vi "BRig_Host_v0,51.vi"() -> ()   [LabVIEW 2014]
uses:
  BRig_Host__global__stopHost.vi
  <vilib>/WebDAVClient/NI_WebDAV.lvlib
  <vilib>/WebDAVClient/Advanced/SessionHandle.ctl
  <vilib>/Utility/file.llb/Write To Spreadsheet File (DBL).vi
panel:
  out "writeError":bool
  out "error IO":errorcluster
  out "error_loopP_loadSettings":errorcluster caption="error out"
  out "testCmdList":u16[][](array[numeric])
  in  "ClosedLoop":bool
  in  "module":string=" module1 "
  in  "input_updateTrial_subsequent":u16
  in  "input_updateTrial_first":u16
  in  "input_forceUpdate":bool
  in  "ClosedLoop":u16[](array[numeric])
  in  "testNewLaserSettings":bool
  in  "LoadSettings":bool
  in  "DisplayNumber":u16
  out "XY Graph":cluster{u16[], u16[]}[](graph)
  in  "threshold_2":u16=600
  in  "threshold_1":u16=300
  in  "Port (F=A/B, T=C)":bool
  out "I_ExpRun":bool
  out "TCP_connection":bool
  in  "stopHost":bool
  # "Port Switch\nToggle TRUE if debugging"
  # "# Trials Displayed\n( 0 = all )"
  # "Selection\nTime Thresholds"
  # "Exp Run\nIn Progress"
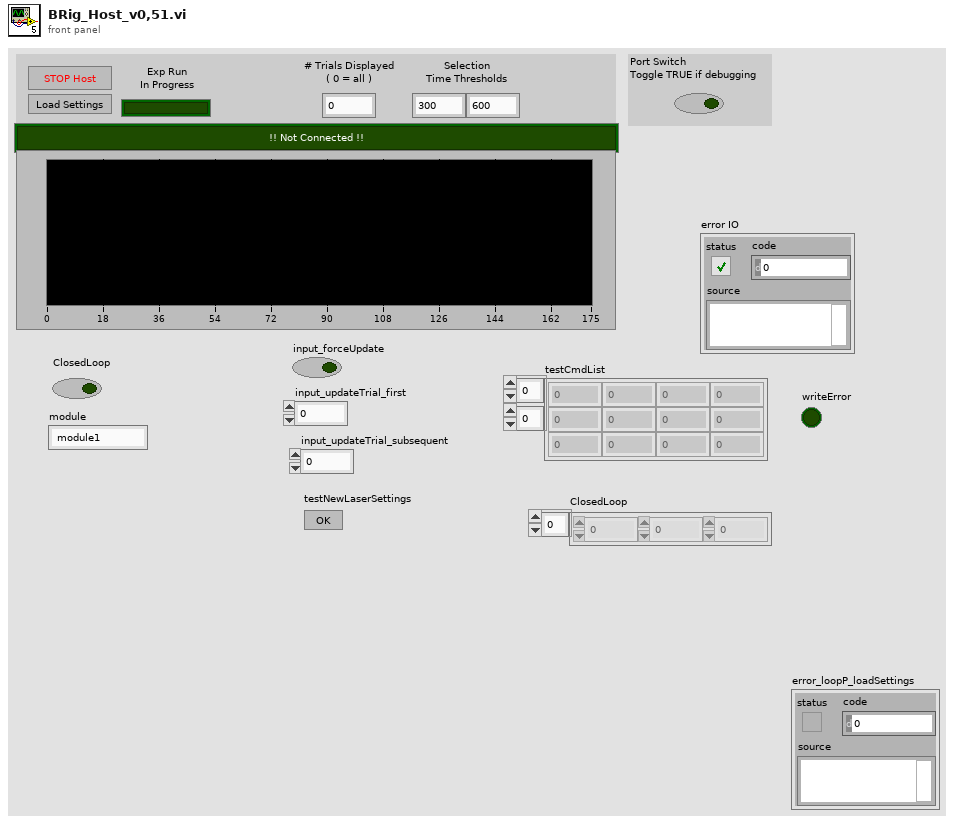
[diagram p1: front panel]
types:
  T1 = typedef "NI_WebDAV.lvlib/SessionHandle.ctl" = refnum<k1>
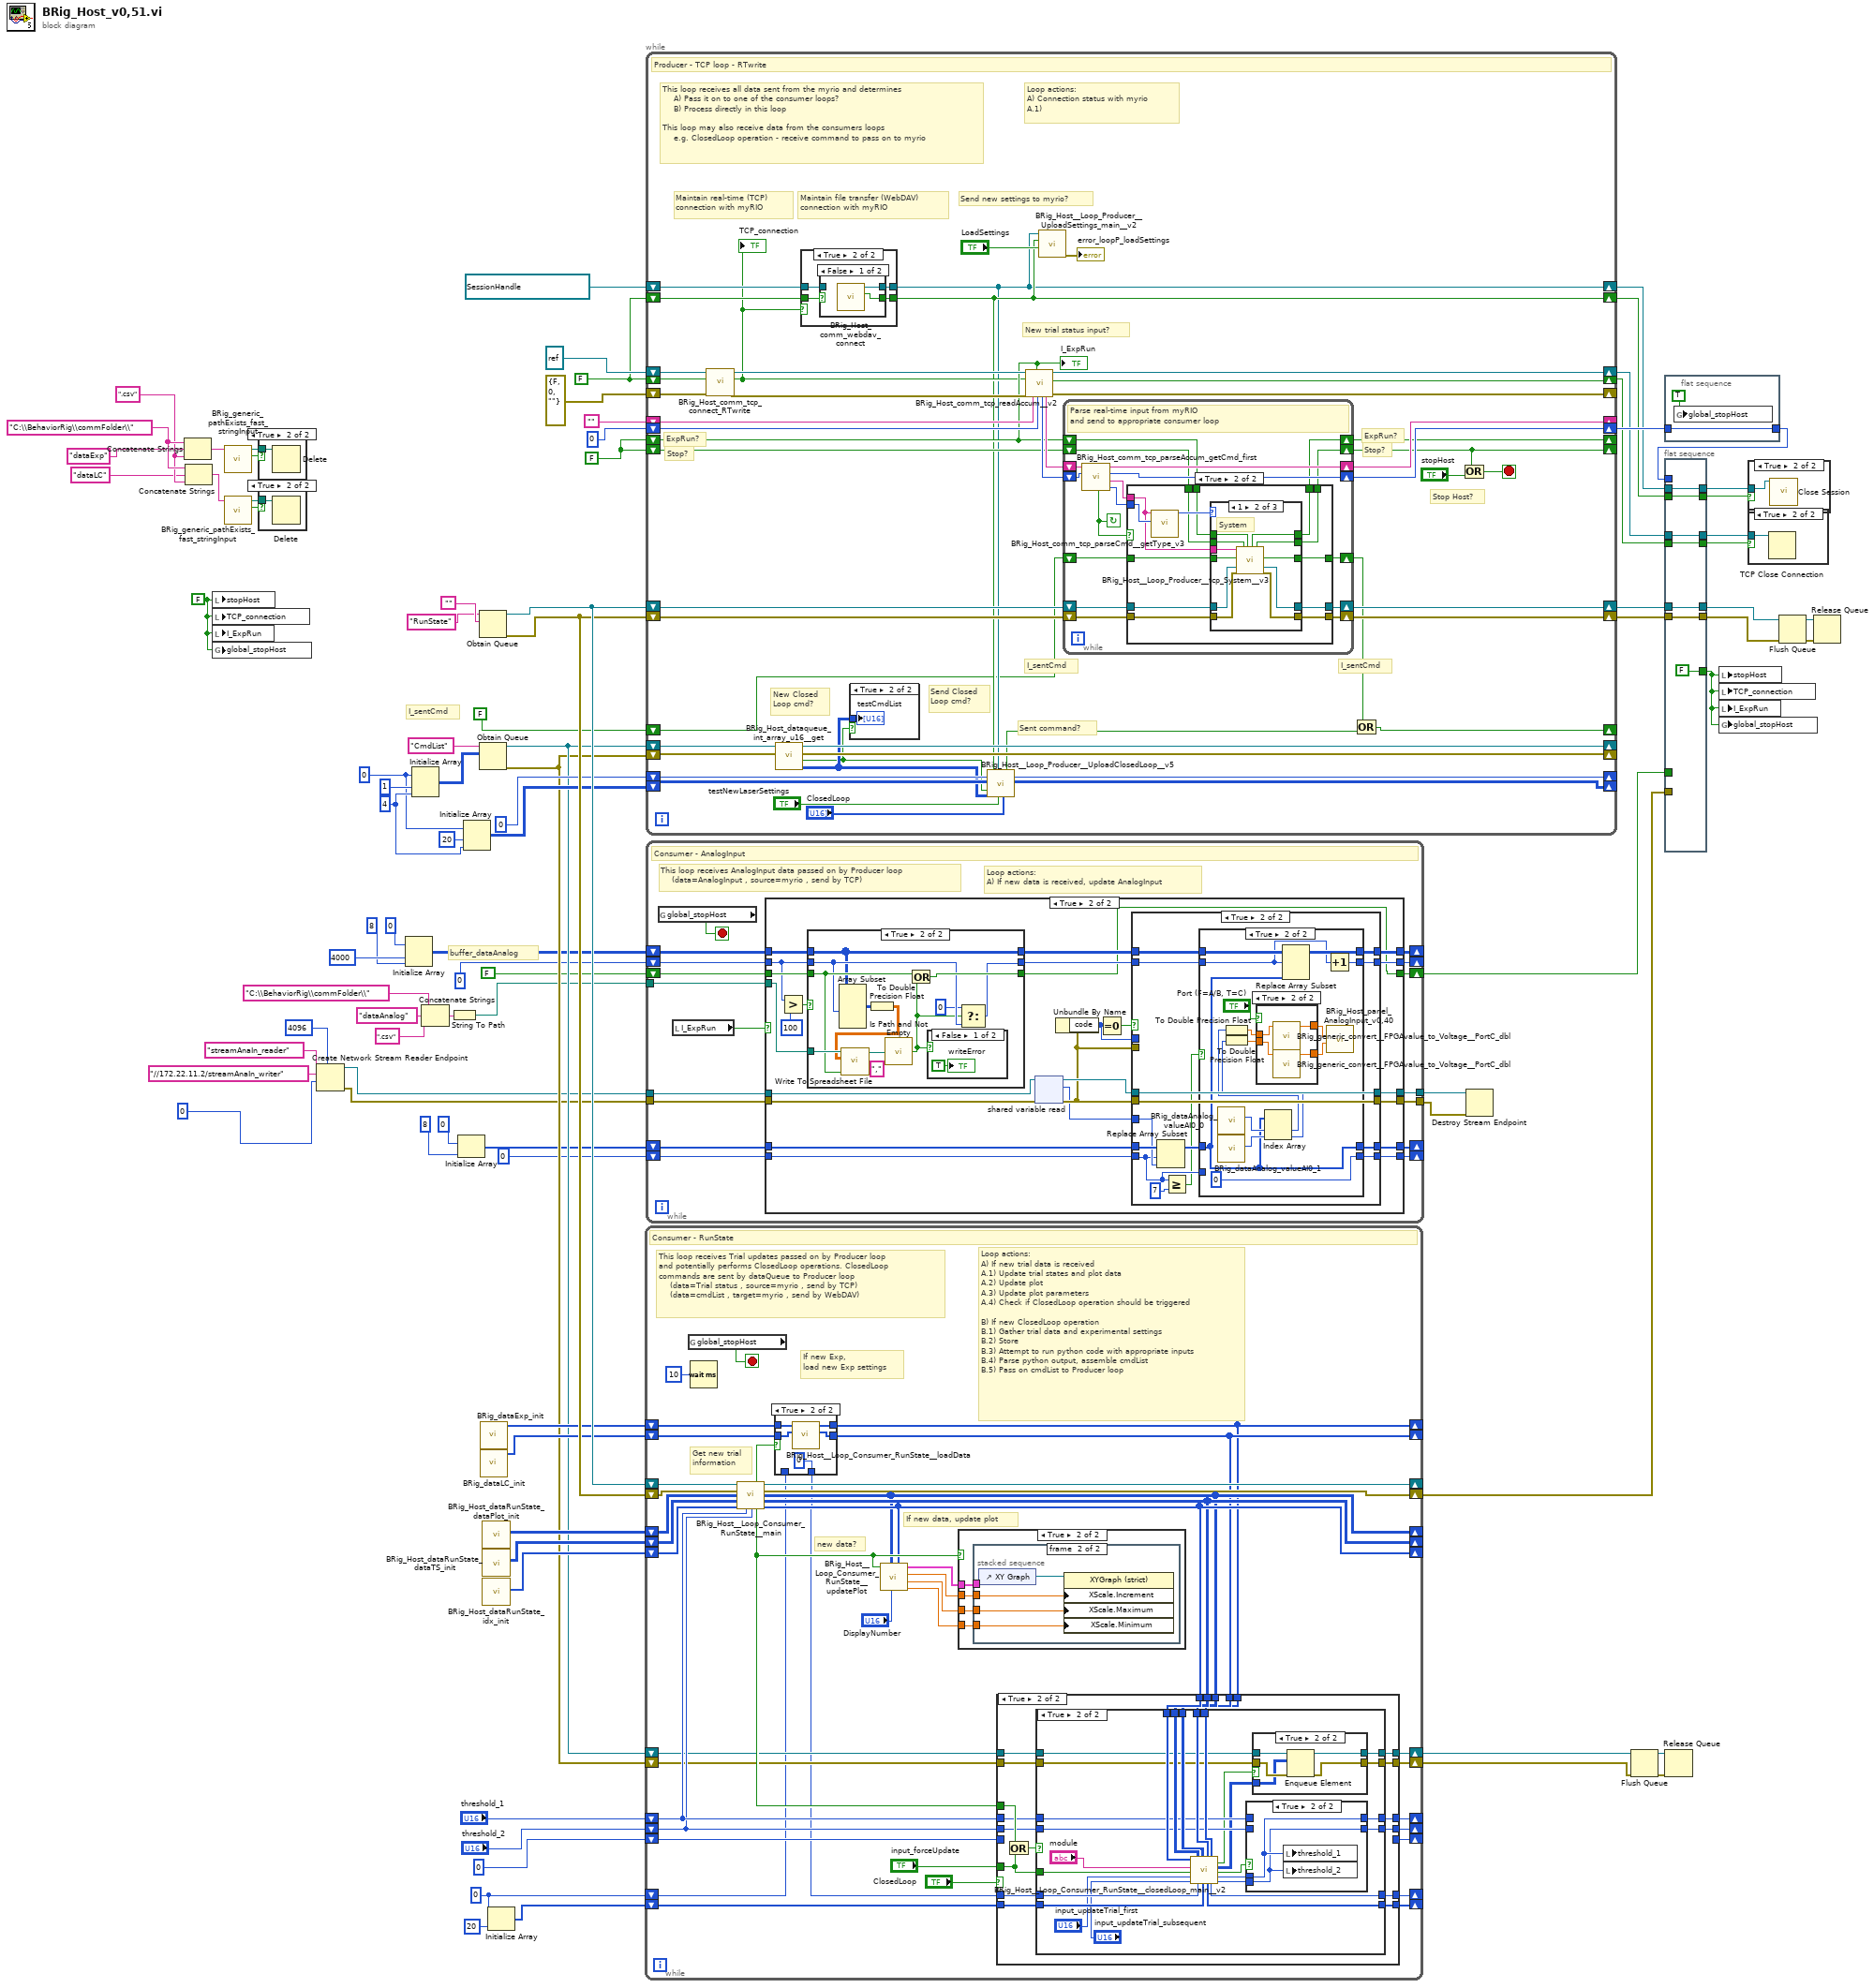
[diagram p0: block diagram]
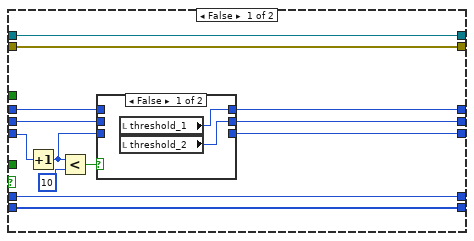
[diagram p6: hidden frame]
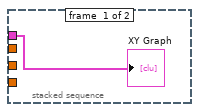
[diagram p13: hidden frame]
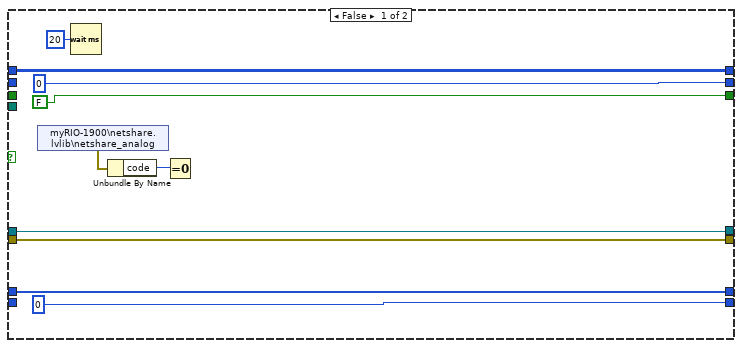
[diagram p14: hidden frame]
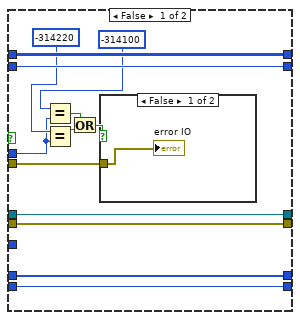
[diagram p15: hidden frame]
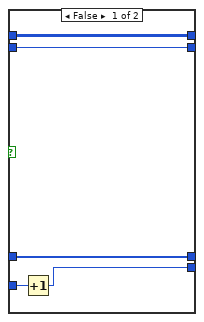
[diagram p17: hidden frame]
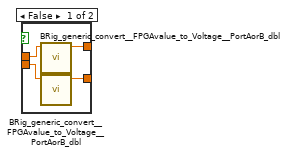
[diagram p18: hidden frame]
diagram:
  w25 = u16 0 ("element")
  w26 = 4 ("dimension size")
  w42 = u16 0
  w54 = ".csv" ("string")
  w55 = "C:\\BehaviorRig\\commFolder\\"
  w67 = T1 refnum items=["Session NI_WebDAV"] ("session handle")
  w85 = FALSE ("stopHost")
  w86 = FALSE
  w68 = FALSE
  # "buffer_dataAnalog"
  # "I_sentCmd"
  n1 = Concatenate Strings(w55, "dataExp" ("string"), w54) -> (w49:string)
  n2 = Concatenate Strings(w55, "dataLC" ("string"), w54) -> (w46:string)
  n3 = local write "stopHost"(w85) -> ()
  n4 = local write "TCP_connection"(w85) -> ()
  n5 = local write "I_ExpRun"(w85) -> ()
  n6 = global write "BRig_Host__global__stopHost.vi" "global_stopHost"(w85) -> ()
  n7 = call "BRig_generic_pathExists_fast_stringInput.vi"("input_filePath"=w49) -> ("output_Iexist"=w51:bool, "output_filePath"=w50:path)  [unwired: 8 in, 1 out]
  n8 = call "BRig_generic_pathExists_fast_stringInput.vi"("input_filePath"=w46) -> ("output_Iexist"=w47:bool, "output_filePath"=w48:path)  [unwired: 8 in, 1 out]
  n9 = case shown="True" w51 {
    tunnel: w50 -> [_ w91]
    frame False {
    }
    frame True {
      n10 = Delete(path (use dialog)=w91) -> ()  [unwired: 4 in, 3 out]
    }
  }
  n11 = case shown="True" w47 {
    tunnel: w48 -> [_ w92]
    frame False {
    }
    frame True {
      n12 = Delete(path (use dialog)=w92) -> ()  [unwired: 4 in, 3 out]
    }
  }
  n13 = Create Network Stream Reader Endpoint(7:4096 ("reader buffer size"), 9:u16 0 ("element"), 10:"//172.22.11.2/streamAnaIn_writer" ("writer url"), 11:"streamAnaIn_reader" ("reader name")) -> (0:w9:errorcluster, 3:w10:refnum<k21>)  [unwired: 3 in]
  n14 = Initialize Array(u16 0 ("element"), 4000 ("dimension size"), 8 ("dimension size")) -> (w21:u16[][])
  n15 = Initialize Array(w25, 1 ("dimension size"), w26) -> (w37:u16[][])
  n16 = Concatenate Strings("C:\\BehaviorRig\\commFolder\\" ("string"), "dataAnalog" ("input_filename"), ".csv" ("string")) -> (w18:string)
  n17 = String To Path(string=w18) -> (path=w15:path)
  n18 = Initialize Array(u16 0 ("element"), 8 ("dimension size")) -> (w2:u16[])
  n19 = Initialize Array(w25, 20 ("dimension size"), w26) -> (w56:u16[][])
  n20 = Obtain Queue(name (unnamed)="RunState", element data type="") -> (queue out=w77:refnum<queue>, error out=w76:errorcluster)  [unwired: 3 in, 1 out]
  n21 = Obtain Queue(name (unnamed)="CmdList", element data type=w37) -> (queue out=w36:refnum<queue>, error out=w35:errorcluster)  [unwired: 3 in, 1 out]
  n22 = call "BRig_dataExp_init.vi"() -> ("output_dataExp"=w45:u16[])  [unwired: 11 in]
  n23 = call "BRig_dataLC_init.vi"() -> ("output_dataLC"=w44:u16[])  [unwired: 11 in]
  n24 = call "BRig_Host_dataRunState_dataPlot_init.vi"() -> ("output_dataPlot"=w73:u16[][])  [unwired: 11 in]
  n25 = call "BRig_Host_dataRunState_dataTS_init.vi"() -> ("output_dataTS"=w72:u16[][])  [unwired: 11 in]
  n26 = call "BRig_Host_dataRunState_idx_init.vi"() -> ("output_idx"=w71:i32[])  [unwired: 11 in]
  n27 = Initialize Array(w42, 20 ("dimension size")) -> (w40:u16[])
  n28 = while {
    shift-right: [w124] -> _
    shift-left: w77 -> [w125]
    shift-right: [w122] -> w30
    shift-left: w76 -> [w123]
    shift-right: [w105] -> _
    shift-left: w73 -> [w121]
    shift-right: [w106] -> _
    shift-left: w72 -> [w120]
    shift-right: [w107] -> _
    shift-left: w71 -> [w119]
    shift-right: [w115] -> _
    shift-left: "threshold_1" -> [w114]
    shift-right: [w113] -> _
    shift-left: "threshold_2" -> [w112]
    shift-right: [w103] -> _
    shift-left: w45 -> [w117]
    shift-right: [w104] -> _
    shift-left: w44 -> [w116]
    shift-right: [w97] -> _
    shift-left: w42 -> [w95]
    shift-right: [w109] -> _
    shift-left: u8 0 -> [w110]
    shift-right: [w96] -> _
    shift-left: w40 -> [w93]
    shift-right: [w100] -> w32
    shift-left: w36 -> [w102]
    shift-right: [w99] -> w31
    shift-left: w35 -> [w101]
    stop <- w132 stop-if-true
    # "Loop actions:\nA) If new trial data is received\nA.1) Update trial states and plot data\nA.2) Update plot\nA.3) Update plot parameters\nA.4) Check if ClosedLoop operation should be triggered\n\nB) If new ClosedLoop operation\nB.1) Gather trial data and experimental settings\nB.2) Store\nB.3) Attempt to run python code with appropriate inputs\nB.4) Parse python output, assemble cmdList\nB.5) Pass on cmdList to Producer loop"
    # "This loop receives Trial updates passed on by Producer loop\nand potentially performs ClosedLoop operations. ClosedLoop\ncommands are sent by dataQueue to Producer loop\n    (data=Trial status , source=myrio , send by TCP)\n    (data=cmdList , target=myrio , send by WebDAV)"
    # "If new data, update plot"
    # "If new Exp,\nload new Exp settings"
    # "new data?"
    # "Get new trial\ninformation"
    # "Consumer - RunState"
    n29 = global read "BRig_Host__global__stopHost.vi" "global_stopHost"() -> (w132:bool)
    n30 = Wait (ms)(milliseconds to wait=u32 10) -> ()  [unwired: 1 out]
    n31 = call "BRig_Host__Loop_Consumer_RunState__main.vi"("input_hDataQueue"=w125, "input_errorDataQueue"=w123, "input_dataPlot"=w121, "input_dataTS"=w120, "input_idx"=w119, "threshold_1"=w114, "threshold_2"=w112) -> ("output_ExpStart"=w118:bool, "output_hDataQueue"=w124:refnum<queue>, "output_errorDataQueue"=w122:errorcluster, "output_dataPlot"=w105:u16[][], "output_dataTS"=w106:u16[][], "output_updatePlot"=w108:bool, "output_idx"=w107:i32[])  [unwired: 2 in]
    n32 = case shown="True" w118 {
      tunnel: w117 -> [w216 w218]
      tunnel: [w216 w221] -> w103
      tunnel: w116 -> [w215 w219]
      tunnel: [w215 w220] -> w104
      tunnel: w95 -> [w214 _]
      tunnel: [w214 u16 0] -> w94
      frame False {
      }
      frame True {
        n33 = call "BRig_Host__Loop_Consumer_RunState__loadData.vi"("input_dataLC"=w219, "input_dataExp"=w218) -> ("output_dataLC"=w220:u16[], "output_dataExp"=w221:u16[])  [unwired: 8 in]
      }
    }
    n34 = call "BRig_Host__Loop_Consumer_RunState__updatePlot.vi"("input_idx"=w107, "input_DisplayNumber"="DisplayNumber", "input_dataPlot"=w105, "input_updatePlot"=w108) -> ("output_X_min"=w128:dbl, "output_X_max"=w127:dbl, "output_X_inc"=w126:dbl, "XY Graph"=w129:cluster{u16[], u16[]}[])  [unwired: 4 in]
    n35 = case shown="True" w108 {
      tunnel: w129 -> [_ w225]
      tunnel: w128 -> [_ w224]
      tunnel: w127 -> [_ w223]
      tunnel: w126 -> [_ w222]
      frame False {
      }
      frame True {
        n36 = stacked-sequence {
          tunnel: w225 -> [w226 _]
          tunnel: w224 -> [_ w229]
          tunnel: w223 -> [_ w228]
          tunnel: w222 -> [_ w227]
          frame #0 {
            "XY Graph" <- w226
          }
          frame #1 {
            n37 = control-ref of="XY Graph"() -> (w230:refnum<vi>)
            n38 = property class="XYGraph (strict)"(reference=w230, "XScale.Increment"=w227, "XScale.Maximum"=w228, "XScale.Minimum"=w229) -> ()  [unwired: 1 in, 2 out]
          }
        }
      }
    }
    n39 = case shown="True" "ClosedLoop" {
      tunnel: [w140 w163] -> w115
      tunnel: w114 -> [w141 w164]
      tunnel: [w139 w161] -> w113
      tunnel: w112 -> [w142 w162]
      tunnel: w110 -> [w145 _]
      tunnel: [w138 _] -> w109
      tunnel: w94 -> [w136 w168]
      tunnel: [w136 w166] -> w97
      tunnel: w93 -> [w135 w167]
      tunnel: [w135 w165] -> w96
      tunnel: w108 -> [_ w170]
      tunnel: w107 -> [_ w160]
      tunnel: w106 -> [_ w159]
      tunnel: w105 -> [_ w158]
      tunnel: w104 -> [_ w157]
      tunnel: w103 -> [_ w156]
      tunnel: w102 -> [w134 w155]
      tunnel: w101 -> [w133 w154]
      tunnel: [w134 w153] -> w100
      tunnel: [w133 w152] -> w99
      tunnel: "input_forceUpdate" -> [_ w151]
      frame False {
        n40 = Increment(x=w145) -> (x+1=w137:u8)
        n41 = Less?(x=w137, y=u8 10) -> (x < y?=w143:bool)
        n42 = case shown="False" w143 {
          tunnel: w142 -> [_ w149]
          tunnel: w141 -> [_ w150]
          tunnel: [w147 w150] -> w140
          tunnel: [w146 w149] -> w139
          tunnel: [_ w148] -> w138
          tunnel: w137 -> [_ w148]
          frame False {
            n43 = local read "threshold_1"() -> (w147:u16)
            n44 = local read "threshold_2"() -> (w146:u16)
          }
          frame True {
          }
        }
      }
      frame True {
        n45 = Or(x=w170, y=w151) -> (x .or. y?=w169:bool)
        n46 = case shown="True" w169 {
          tunnel: w151 -> [_ w199]
          tunnel: w168 -> [w176 w202]
          tunnel: w167 -> [w175 w201]
          tunnel: [w176 w195] -> w166
          tunnel: [w175 w196] -> w165
          tunnel: w164 -> [w174 w189]
          tunnel: [w174 w185] -> w163
          tunnel: w162 -> [w173 w188]
          tunnel: [w173 w184] -> w161
          tunnel: w160 -> [_ w194]
          tunnel: w159 -> [_ w193]
          tunnel: w158 -> [_ w192]
          tunnel: w157 -> [_ w191]
          tunnel: w156 -> [_ w190]
          tunnel: w155 -> [w172 w182]
          tunnel: w154 -> [w171 w180]
          tunnel: [w172 w181] -> w153
          tunnel: [w171 w179] -> w152
          frame False {
          }
          frame True {
            n47 = call "BRig_Host__Loop_Consumer_RunState__closedLoop_main__v2.vi"("input_idx"=w194, "input_module"="module", "input_forceUpdate"=w199, "input_updateTrial_first"="input_updateTrial_first", "input_updateTrial_subsequent"="input_updateTrial_subsequent", "input_dataTS"=w193, "input_updateID"=w202, "input_dataPlot"=w192, "input_trialList"=w201, "input_dataLC"=w191, "input_dataExp"=w190) -> ("output_trialList"=w196:u16[], "output_updateID"=w195:u16, 15:"output_cmdList"=w177:bool, 16:"output_cmdList"=w178:u16[][], "output_thres"=w183:bool, "output_thres1"=w187:u16, "output_thres2"=w186:u16)  [unwired: 2 in]
            n48 = case shown="True" w183 {
              tunnel: w189 -> [w211 _]
              tunnel: w188 -> [w210 _]
              tunnel: w187 -> [_ w213]
              tunnel: w186 -> [_ w212]
              tunnel: [w211 w213] -> w185
              tunnel: [w210 w212] -> w184
              frame False {
              }
              frame True {
                n49 = local write "threshold_1"(w213) -> ()
                n50 = local write "threshold_2"(w212) -> ()
              }
            }
            n51 = case shown="True" w177 {
              tunnel: w182 -> [w204 w209]
              tunnel: [w204 w206] -> w181
              tunnel: w180 -> [w203 w208]
              tunnel: [w203 w205] -> w179
              tunnel: w178 -> [_ w207]
              frame False {
              }
              frame True {
                n52 = Enqueue Element(queue=w209, element=w207, error in (no error)=w208) -> (queue out=w206:refnum<queue>, error out=w205:errorcluster)  [unwired: 1 in, 1 out]
              }
            }
          }
        }
      }
    }
  }
  n53 = while {
    shift-right: [w257] -> w61
    shift-left: w68 -> [w277]
    shift-right: [w272] -> w62
    shift-left: refnum<k5> refnum ("output_hTCP") -> [w276]
    shift-right: [w271] -> _
    shift-left: errorcluster {"status"=FALSE, "code"=0, "source"=""} ("output_error") -> [w275]
    shift-right: [w266] -> _
    shift-left: "" ("input_strAccum") -> [w270]
    shift-right: [w265] -> w75
    shift-left: 0 ("input_count") -> [w269]
    shift-right: [w264] -> _
    shift-left: w86 -> [w242]
    shift-right: [w240] -> _
    shift-left: w86 -> [w262]
    shift-right: [w259] -> w81
    shift-left: w77 -> [w261]
    shift-right: [w258] -> w80
    shift-left: w76 -> [w260]
    shift-right: [w237] -> w66
    shift-left: w68 -> [w256]
    shift-right: [w236] -> w65
    shift-left: w67 -> [w255]
    shift-right: [w247] -> _
    shift-left: w56 -> [w248]
    shift-right: [w231] -> _
    shift-left: 0 -> [w249]
    shift-right: [w251] -> _
    shift-left: w36 -> [w253]
    shift-right: [w250] -> _
    shift-left: w35 -> [w252]
    shift-right: [w232] -> _
    shift-left: FALSE -> [w235]
    stop <- w239 stop-if-true
    # "Sent command?"
    # "I_sentCmd"
    # "I_sentCmd"
    # "Stop Host?"
    # "Send Closed\nLoop cmd?"
    # "New Closed\nLoop cmd?"
    # "New trial status input?"
    # "ExpRun?"
    # "Stop?"
    # "Loop actions:\nA) Connection status with myrio\nA.1)"
    # "This loop receives all data sent from the myrio and determines\n    A) Pass it on to one of the consumer loops?\n    B) Process directly in this loop\n\nThis loop may also receive data from the consumers loops\n    e.g. ClosedLoop operation - receive command to pass on to myrio"
    # "Send new settings to myrio?"
    # "ExpRun?"
    # "Stop?"
    # "Maintain real-time (TCP)\nconnection with myRIO"
    # "Maintain file transfer (WebDAV)\nconnection with myRIO"
    # "Producer - TCP loop - RTwrite"
    n54 = call "BRig_Host_comm_tcp_connect_RTwrite.vi"("input_error"=w275, "input_connected"=w277, "input_hTCP"=w276) -> ("output_error"=w273:errorcluster, "output_connected"=w241:bool, "output_hTCP"=w274:refnum<k5>)  [unwired: 5 in, 1 out]
    "TCP_connection" <- w241
    n55 = call "BRig_Host_dataqueue_int_array_u16__get.vi"("input_erroDataQueue"=w252, "input_hDataQueue"=w253) -> (0:"output_data"=w244:u16[][], 1:"output_data"=w243:bool, "output_errorDataQueue"=w250:errorcluster, "output_hDataQueue"=w251:refnum<queue>)  [unwired: 6 in]
    n56 = case shown="True" w241 {
      tunnel: w256 -> [w282 w290]
      tunnel: [w281 w289] -> w237
      tunnel: w255 -> [w280 w288]
      tunnel: [w279 w287] -> w236
      frame False {
        n57 = case shown="True" w282 {
          selector: w282 -> [w284 _]
          tunnel: [w284 FALSE] -> w281
          tunnel: w280 -> [w283 w285]
          tunnel: [w283 _] -> w279
          frame False {
          }
          frame True {
            n58 = call <vilib>:"Close Session.vi"("session handle"=w285) -> ()  [unwired: 14 in, 1 out]
          }
        }
      }
      frame True {
        n59 = case shown="False" w290 {
          selector: w290 -> [_ w294]
          tunnel: [w291 w294] -> w289
          tunnel: w288 -> [_ w293]
          tunnel: [w292 w293] -> w287
          frame False {
            n60 = call "BRig_Host_comm_webdav_connect.vi"() -> ("output_Iconnected"=w291:bool, "output_hSession"=w292:T1)  [unwired: 9 in, 1 out]
          }
          frame True {
          }
        }
      }
    }
    n61 = case shown="True" w243 {
      tunnel: w244 -> [_ w278]
      frame False {
      }
      frame True {
        "testCmdList" <- w278
      }
    }
    n62 = call "BRig_Host__Loop_Producer__UploadClosedLoop__v5.vi"("input_arrayBuffer_length"=w249, "input_arrayBuffer"=w248, 4:"input_cmdList"=w243, 5:"input_cmdList"=w244, "input_webdav_status"=w237, "session handle"=w236, "testNewLaserSettings"="testNewLaserSettings", "input_array_LaserSettings"="ClosedLoop") -> ("Sent"=w233:bool, "output_arrayBuffer_length"=w231:i32, "output_arrayBuffer"=w247:u16[][])  [unwired: 9 in]
    n63 = call "BRig_Host_comm_tcp_readAccum__v2.vi"("input_handle_TCP"=w274, "input_connected"=w241, "input_error"=w273, "input_strAccum"=w270, "input_I_ExpRun"=w242, "input_count"=w269) -> ("output_count"=w267:i32, "output_strAccum"=w268:string, "output_handle_TCP"=w272:refnum<k5>, "output_connected"=w257:bool, "output_error"=w271:errorcluster)  [unwired: 9 in]
    n64 = call "BRig_Host__Loop_Producer__UploadSettings_main__v2.vi"("input_LoadSettings"="LoadSettings", "input_webdav_status"=w237, "session handle"=w236) -> ("error out"=→"error_loopP_loadSettings":errorcluster)  [unwired: 8 in]
    n65 = while {
      shift-right: [w308] -> w266
      shift-left: w268 -> [w311]
      shift-right: [w307] -> w265
      shift-left: w267 -> [w310]
      shift-right: [w303] -> w264
      shift-left: w242 -> [w304]
      shift-right: [w301] -> w240
      shift-left: w262 -> [w302]
      shift-right: [w297] -> w259
      shift-left: w261 -> [w300]
      shift-right: [w298] -> w258
      shift-left: w260 -> [w299]
      shift-right: [w295] -> w234
      shift-left: w235 -> [w296]
      stop <- w309 continue-if-true
      # "Parse real-time input from myRIO\nand send to appropriate consumer loop"
      n66 = call "BRig_Host_comm_tcp_parseAccum_getCmd_first.vi"("input_count"=w310, "input_strAccum"=w311) -> ("output_countCmd"=w305:i32, "output_strCmd"=w306:string, "output_count"=w307:i32, "output_strAccum"=w308:string, "output_I_cmd"=w309:bool)  [unwired: 5 in]
      n67 = case shown="True" w309 {
        tunnel: w306 -> [_ w327]
        tunnel: w305 -> [_ w329]
        tunnel: w304 -> [w316 w322]
        tunnel: [w316 w320] -> w303
        tunnel: w302 -> [w315 w321]
        tunnel: [w315 w319] -> w301
        tunnel: w300 -> [w314 w326]
        tunnel: w299 -> [w313 w325]
        tunnel: [w313 w324] -> w298
        tunnel: [w314 w323] -> w297
        tunnel: w296 -> [w312 w318]
        tunnel: [w312 w317] -> w295
        frame False {
        }
        frame True {
          n68 = call "BRig_Host_comm_tcp_parseCmd__getType_v3.vi"("input_strCmd"=w327, "input_countCmd"=w329) -> ("output_strType"=w328:u8)  [unwired: 17 in]
          n69 = case shown="1" w328 {
            tunnel: w327 -> [_ w341 w353]
            tunnel: w326 -> [w334 w344 w352]
            tunnel: w325 -> [w333 w345 w351]
            tunnel: [w333 w343 w350] -> w324
            tunnel: [w334 w342 w349] -> w323
            tunnel: w322 -> [w332 w340 w348]
            tunnel: w321 -> [w331 w339 w347]
            tunnel: [w332 w338 w348] -> w320
            tunnel: [w331 w337 w347] -> w319
            tunnel: w318 -> [w330 w336 w346]
            tunnel: [w330 w335 w346] -> w317
            frame 0, Default {
            }
            frame 1 {
              # "System"
              n70 = call "BRig_Host__Loop_Producer__tcp_System__v3.vi"("input_strCmd"=w341, "input_I_SentCmd"=w336, "input_hDataQueue"=w344, "input_error_dataqueue"=w345, "input_I_Stop"=w339, "input_I_ExpRun"=w340) -> ("output_I_ExpRun"=w338:bool, "output_I_Stop"=w337:bool, "output_I_sentCmd"=w335:bool, "output_hDataQueue"=w342:refnum<queue>, "output_error"=w343:errorcluster)  [unwired: 9 in]
            }
            frame 2 {
              # "RunState"
              n71 = Enqueue Element(queue=w352, element=w353, error in (no error)=w351) -> (queue out=w349:refnum<queue>, error out=w350:errorcluster)  [unwired: 1 in, 1 out]
            }
          }
        }
      }
    }
    n72 = Or(x=w234, y=w233) -> (x .or. y?=w232:bool)
    n73 = Or(x=w240, y="stopHost") -> (x .or. y?=w239:bool)
    "I_ExpRun" <- w242
  }
  n74 = while {
    shift-right: [w367] -> _
    shift-left: w21 -> [w369]
    shift-right: [w366] -> _
    shift-left: 0 -> [w368]
    tunnel: w15 -> [w365]
    shift-right: [w363] -> w13
    shift-left: FALSE -> [w364]
    tunnel: w10 -> [w361]
    tunnel: w9 -> [w360]
    tunnel: [w359] -> w7
    tunnel: [w358] -> w6
    shift-right: [w355] -> _
    shift-left: w2 -> [w357]
    shift-right: [w354] -> _
    shift-left: 0 ("element") -> [w356]
    stop <- w370 stop-if-true
    # "Loop actions:\nA) If new data is received, update AnalogInput"
    # "This loop receives AnalogInput data passed on by Producer loop\n    (data=AnalogInput , source=myrio , send by TCP)"
    # "Consumer - AnalogInput"
    n75 = global read "BRig_Host__global__stopHost.vi" "global_stopHost"() -> (w370:bool)
    n76 = local read "I_ExpRun"() -> (w362:bool)
    n77 = case shown="True" w362 {
      tunnel: w369 -> [w377 w403]
      tunnel: w368 -> [_ w389]
      tunnel: [w377 w398] -> w367
      tunnel: [0 w396] -> w366
      tunnel: w365 -> [_ w401]
      tunnel: w364 -> [_ w402]
      tunnel: [FALSE w386] -> w363
      tunnel: w361 -> [w374 w395]
      tunnel: w360 -> [w373 w394]
      tunnel: [w374 w392] -> w359
      tunnel: [w373 w390] -> w358
      tunnel: w357 -> [w372 w384]
      tunnel: w356 -> [_ w383]
      tunnel: [w372 w382] -> w355
      tunnel: [0 ("element") w381] -> w354
      frame False {
        n78 = shared-variable "myRIO-1900\\netshare.lvlib\\netshare_analog"() -> (error out=w379:errorcluster)  [unwired: 1 in, 1 out]
        n79 = Wait (ms)(milliseconds to wait=u32 20) -> ()  [unwired: 1 out]
        n80 = Unbundle By Name(w379) -> ("code"=w378:i32)
        n81 = Equal To 0?(x=w378) -> ()  [unwired: 1 out]
      }
      frame True {
        n82 = Greater?(x=w389, y=100) -> (0:w404:bool)
        n83 = case shown="True" w404 {
          tunnel: w403 -> [w463 w466]
          tunnel: [w463 w466] -> w399
          tunnel: w389 -> [w462 w468]
          tunnel: w402 -> [w461 w470]
          tunnel: [w462 w467] -> w397
          tunnel: [w461 w469] -> w386
          tunnel: w401 -> [_ w475]
          frame False {
          }
          frame True {
            n84 = Array Subset(array=w466, length (row)=w468) -> (w474:u16[][])  [unwired: 3 in]
            n85 = To Double Precision Float(number=w474) -> (double precision float=w473:dbl[][])
            n86 = call-poly <vilib>:"Write To Spreadsheet File.vi"("delimiter (\\t)"="," ("delimiter (\\t)"), "append to file? (new file:F)"=w470, "2D data"=w473, "file path (dialog if empty)"=w475) -> ("new file path (Not A Path if cancelled)"=w471:path)  [unwired: 4 in]
            n87 = call <vilib>:"Is Path and Not Empty.vi"("path"=w471) -> ("Is Path and Not Empty?"=w464:bool)  [unwired: 4 in]
            n88 = Or(x=w470, y=w464) -> (x .or. y?=w469:bool)
            n89 = case shown="False" w464 {
              frame False {
                "writeError" <- TRUE ("writeError")
              }
              frame True {
              }
            }
            n90 = Select(t=0, s=w464, f=w468) -> (s? t:f=w467:i32)
          }
        }
        n91 = shared-variable-read(w395, w394) -> (w393:refnum<k21>, w391:errorcluster, w385:u16)  [unwired: 1 in, 1 out]
        n92 = Unbundle By Name(w391) -> ("code"=w387:i32)
        n93 = Equal To 0?(x=w387) -> (x = 0?=w400:bool)
        n94 = case shown="True" w400 {
          tunnel: w399 -> [w417 w432]
          tunnel: [w417 w431] -> w398
          tunnel: w397 -> [w416 w430]
          tunnel: [w416 w429] -> w396
          tunnel: w391 -> [w414 _]
          tunnel: w393 -> [w413 w428]
          tunnel: [w413 w428] -> w392
          tunnel: w391 -> [w412 w427]
          tunnel: [w412 w427] -> w390
          tunnel: w387 -> [w411 _]
          tunnel: w385 -> [_ w425]
          tunnel: w384 -> [w406 w426]
          tunnel: w383 -> [w405 w423]
          tunnel: [w406 w420] -> w382
          tunnel: [w405 w422] -> w381
          frame False {
            n95 = Equal?(x=-314100, y=w411) -> (x = y?=w409:bool)
            n96 = Equal?(x=-314220, y=w411) -> (x = y?=w408:bool)
            n97 = Or(x=w409, y=w408) -> (x .or. y?=w407:bool)
            n98 = case shown="False" w407 {
              tunnel: w414 -> [w418 _]
              frame False {
                "error IO" <- w418
              }
              frame True {
              }
            }
          }
          frame True {
            n99 = Replace Array Subset(array=w426, new element=w425, index=w423) -> (w421:u16[])
            n100 = Greater Or Equal?(x=w423, y=7) -> (x >= y?=w419:bool)
            n101 = case shown="True" w419 {
              tunnel: w432 -> [w437 w452]
              tunnel: [w437 w451] -> w431
              tunnel: w430 -> [w436 w450]
              tunnel: [w436 w449] -> w429
              tunnel: w423 -> [w435 _]
              tunnel: [w434 0 ("y")] -> w422
              tunnel: w421 -> [w433 w440]
              tunnel: [w433 w440] -> w420
              frame False {
                n102 = Increment(x=w435) -> (x+1=w434:i32)
              }
              frame True {
                n103 = call "BRig_dataAnalog_valueAI0_0.vi"() -> ("output_valueAI0_0"=w442:i32)  [unwired: 11 in]
                n104 = call "BRig_dataAnalog_valueAI0_1.vi"() -> ("output_valueAI0_1"=w443:i32)  [unwired: 11 in]
                n105 = Index Array(array=w440, index #1=w442, index #2=w443) -> (element #1=w439:u16, element #2=w438:u16)
                n106 = To Double Precision Float(number=w439) -> (double precision float=w444:dbl)
                n107 = To Double Precision Float(number=w438) -> (double precision float=w445:dbl)
                n108 = case shown="True" "Port (F=A/B, T=C)" {
                  tunnel: w444 -> [w454 w460]
                  tunnel: w445 -> [w453 w459]
                  tunnel: [w456 w458] -> w447
                  tunnel: [w455 w457] -> w446
                  frame False {
                    n109 = call "BRig_generic_convert__FPGAvalue_to_Voltage__PortAorB_dbl.vi"("input_FPGAvalue_PortAorB"=w454) -> ("output_voltage"=w456:dbl)  [unwired: 10 in]
                    n110 = call "BRig_generic_convert__FPGAvalue_to_Voltage__PortAorB_dbl.vi"("input_FPGAvalue_PortAorB"=w453) -> ("output_voltage"=w455:dbl)  [unwired: 10 in]
                  }
                  frame True {
                    n111 = call "BRig_generic_convert__FPGAvalue_to_Voltage__PortC_dbl.vi"("input_FPGAvalue_PortC"=w460) -> ("output_voltage"=w458:dbl)  [unwired: 10 in]
                    n112 = call "BRig_generic_convert__FPGAvalue_to_Voltage__PortC_dbl.vi"("input_FPGAvalue_PortC"=w459) -> ("output_voltage"=w457:dbl)  [unwired: 10 in]
                  }
                }
                n113 = Replace Array Subset(array=w452, new element=w440, index (row)=w450) -> (w451:u16[][])  [unwired: 1 in]
                n114 = Increment(x=w450) -> (x+1=w449:i32)
                n115 = call "BRig_Host_panel_AnalogInput_v0,40.vi"("graph_ai1"=w446, "graph_ai0"=w447) -> ()  [unwired: 10 in]
              }
            }
          }
        }
      }
    }
  }
  n116 = Destroy Stream Endpoint(8:w6, 11:w7) -> ()  [unwired: 1 out]
  n117 = Flush Queue(queue=w32, error in (no error)=w31) -> (queue out=w34:refnum<queue>, error out=w33:errorcluster)  [unwired: 1 out]
  n118 = flat-sequence {
    tunnel: w75 -> [w477]
    tunnel: [w477] -> w74
    frame #0 {
      n119 = global write "BRig_Host__global__stopHost.vi" "global_stopHost"(TRUE ("global_stopHost")) -> ()
    }
  }
  n120 = flat-sequence {
    tunnel: [FALSE] -> w84
    tunnel: w81 -> [w484]
    tunnel: w80 -> [w483]
    tunnel: [w484] -> w79
    tunnel: [w483] -> w78
    tunnel: w74 -> [_]
    tunnel: w66 -> [w481]
    tunnel: w65 -> [w482]
    tunnel: [w482] -> w63
    tunnel: [w481] -> w64
    tunnel: w62 -> [w479]
    tunnel: w61 -> [w480]
    tunnel: [w480] -> w60
    tunnel: [w479] -> w59
    tunnel: w30 -> [_]
    tunnel: w13 -> [_]
    frame #0 {
    }
  }
  n121 = Release Queue(queue=w34, error in (no error)=w33) -> ()  [unwired: 1 in, 3 out]
  n122 = local write "stopHost"(w84) -> ()
  n123 = local write "TCP_connection"(w84) -> ()
  n124 = local write "I_ExpRun"(w84) -> ()
  n125 = global write "BRig_Host__global__stopHost.vi" "global_stopHost"(w84) -> ()
  n126 = case shown="True" w64 {
    tunnel: w63 -> [_ w486]
    frame False {
    }
    frame True {
      n127 = call <vilib>:"Close Session.vi"("session handle"=w486) -> ()  [unwired: 14 in, 1 out]
    }
  }
  n128 = case shown="True" w60 {
    tunnel: w59 -> [_ w487]
    frame False {
    }
    frame True {
      n129 = TCP Close Connection(connection ID=w487) -> ()  [unwired: 2 in, 2 out]
    }
  }
  n130 = Flush Queue(queue=w79, error in (no error)=w78) -> (queue out=w29:refnum<queue>, error out=w28:errorcluster)  [unwired: 1 out]
  n131 = Release Queue(queue=w29, error in (no error)=w28) -> ()  [unwired: 1 in, 3 out]
